vi "o3 Serial Data Recording & DECADEv3.1(serial_sim).vi"() -> ()   [LabVIEW 2014]
uses:
  <vilib>/Platform/TimedLoop/XDataNode/timing_clust.ctl
  <vilib>/Platform/TimedLoop/XDataNode/nitl_modes.ctl
  <vilib>/Platform/TimedLoop/XDataNode/wakeup.ctl
  C:/Program Files (x86)/National Instruments/LabVIEW 2014/examples/Data Communication/Network Streams/Simple Network Streams/support/Network Stream Command.ctl
  <vilib>/Utility/error.llb/whitespace.ctl
  <vilib>/Utility/tcp.llb/UDP Multicast Read-Only Open.vi
  <vilib>/Utility/tcp.llb/UDP Multicast Write-Only Open.vi
  <vilib>/platform/TimedLoop/XDataNode/XDataNode.xnode
  <vilib>/Platform/TimedLoop/XDataNode/XDNodeRunTimeDep.lvlib
  <vilib>/Instr/_visa.llb/VISA Configure Serial Port (Instr).vi
panel:
  out "error out":errorcluster
  out "V6":bool
  in  "Clear Display\nErrors":bool
  out "Data Processing":bool
  out "Serial Visa Error":errorcluster
  out "SEPTIC TCP Error Out":errorcluster
  out "TCP packet\nSend to SEPTIC":bool
  in  "Time Stamp\nOffset":u32=1
  out "UDP_In_Error":errorcluster
  out "UDP_In":string
  out "Data Array":string[](array[string])
  out "UDP packet \nstatus":bool
  out "UDP_Out_Error":errorcluster
  out "FISH TCP Error Out":errorcluster
  out "TCP packet\nSend to FISH":bool
  out "TCP Binary Packet":string
  out "Scan from String Error Counter\nfrom process loop":i32
  out "Read Error Counter\nfrom process loop":i32
  in  "milliseconds to wait":u32=330
  in  "ID":string="±"
  in  "VISA resource name":refnum<visa-resource-name>="ASRL6::INSTR"
  out "Data In Array":string[](array[string])
  out "UDP_ASCII_Out":string
  out "UDP_Pack_num":u32
  in  "Flight Number":string
  in  "aux":string="0"
  in  "inlet_overq_mfm":string="0"
  in  "acs2653pc_hdd":string="0"
  in  "LabviewVIclient vn":string="0"
  in  "LabviewVIserver vn":string="0"
  in  "acs2653pc temp":string="0"
  in  "ue9LJ temp":u16
  in  "PTP Sync":string="0"
  out "Data String":string
  out "Internal packet":string[](array[string])
  out "RAW DATA":string
  in  "stop":bool
  out "Number of Send & Read Error\nfrom Acquire Loop":i32
  out "Command In":string
  # "o3_conc"
  # "Bench_temp"
  # "pressure"
  # "cell_a_nt"
  # "cell_b_int"
  # "flow_a"
  # "flow_b"
  # "lamp_temp"
  # "flags"
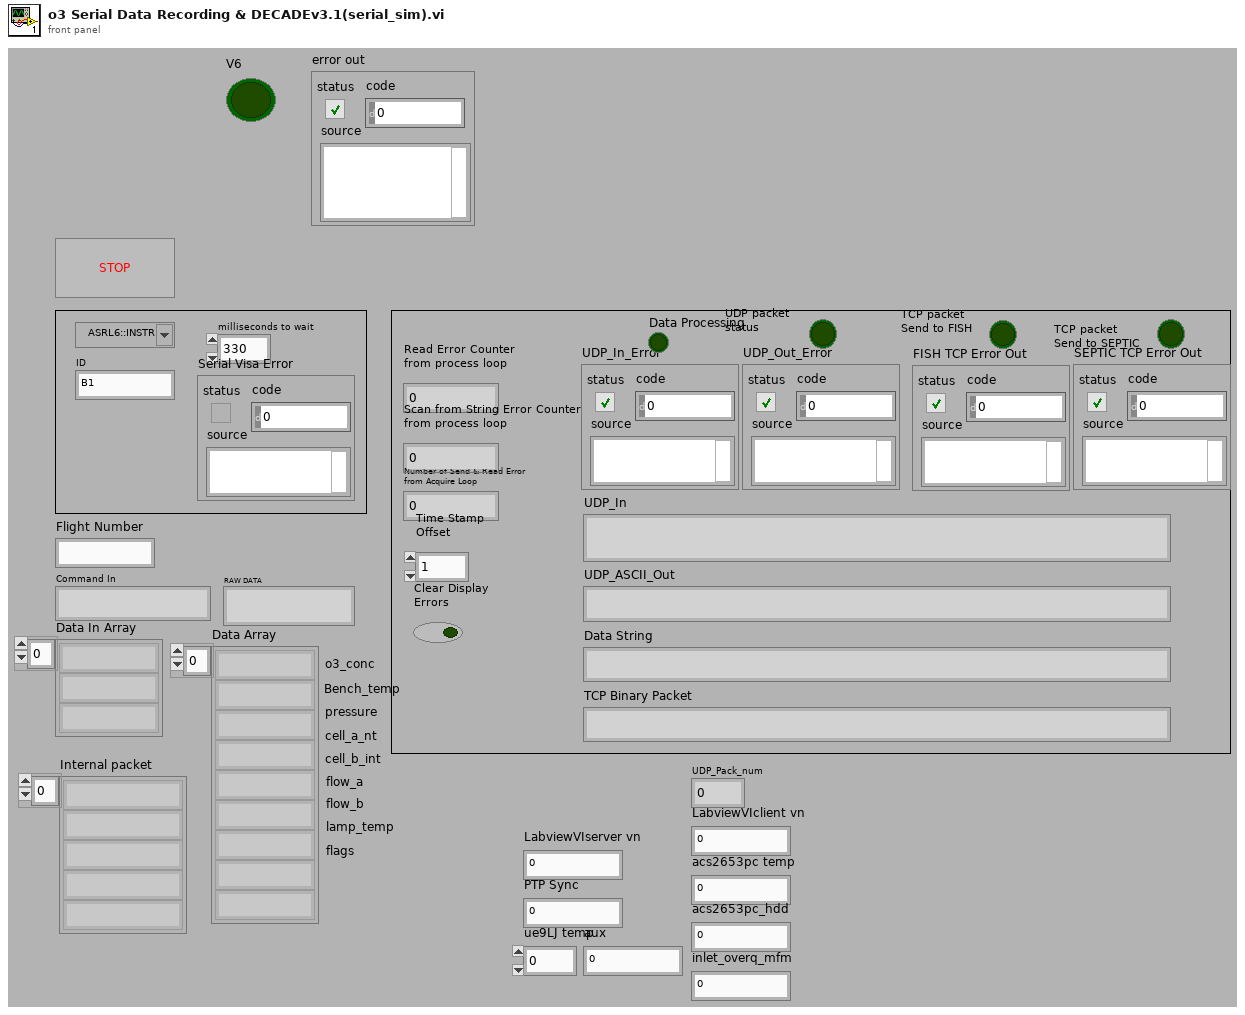
[diagram p1: front panel]
types:
  T1 = typedef "Network Stream Command.ctl" = cluster{"Message":string, "Message Data":variant}
  T2 = typedef "XDNodeRunTimeDep.lvlib/timing_clust.ctl" = cluster{"Expected End [f-1]":u64, "Actual End [f-1]":u64, "Finished Late? [f-1]":bool, "Expected End [i-1]":u64, "Actual End [i-1]":u64, "Finished Late? [i-1]":bool, "Expected Start [i]":u64, "Actual Start [i]":u64, "Expected Start [f]":u64, "Actual Start [f]":u64, "Source Name":string, "Structure Name":string, "Period":i64, "Deadline":i64, "Offset":i64, "Start":i64, "Priority":i32, "Timeout":i32, "Mode":T3, "Wakeup Reason":T4, "Error":errorcluster, "Source Type":string, "Secondary Source Type":string, "Global End Time":u64, "Global Start Time":u64, "Frame Duration":u64, "Iteration Duration":u64, "Assigned CPU":i32, "I/O Scan Engine Mode":u32}
  T3 = typedef "XDNodeRunTimeDep.lvlib/nitl_modes.ctl" = enum32{"No Change", "Process missed periods, maintain original phase", "Discard missed periods, maintain original phase", "Process missed periods, ignore original phase", "Discard missed periods, ignore original phase"}
  T4 = typedef "XDNodeRunTimeDep.lvlib/wakeup.ctl" = enum32{"Normal", "Aborted", "Asynchronous wakeup", "Timing source error", "Timed loop error", "Timeout"}
  T5 = typedef "whitespace.ctl" = u16
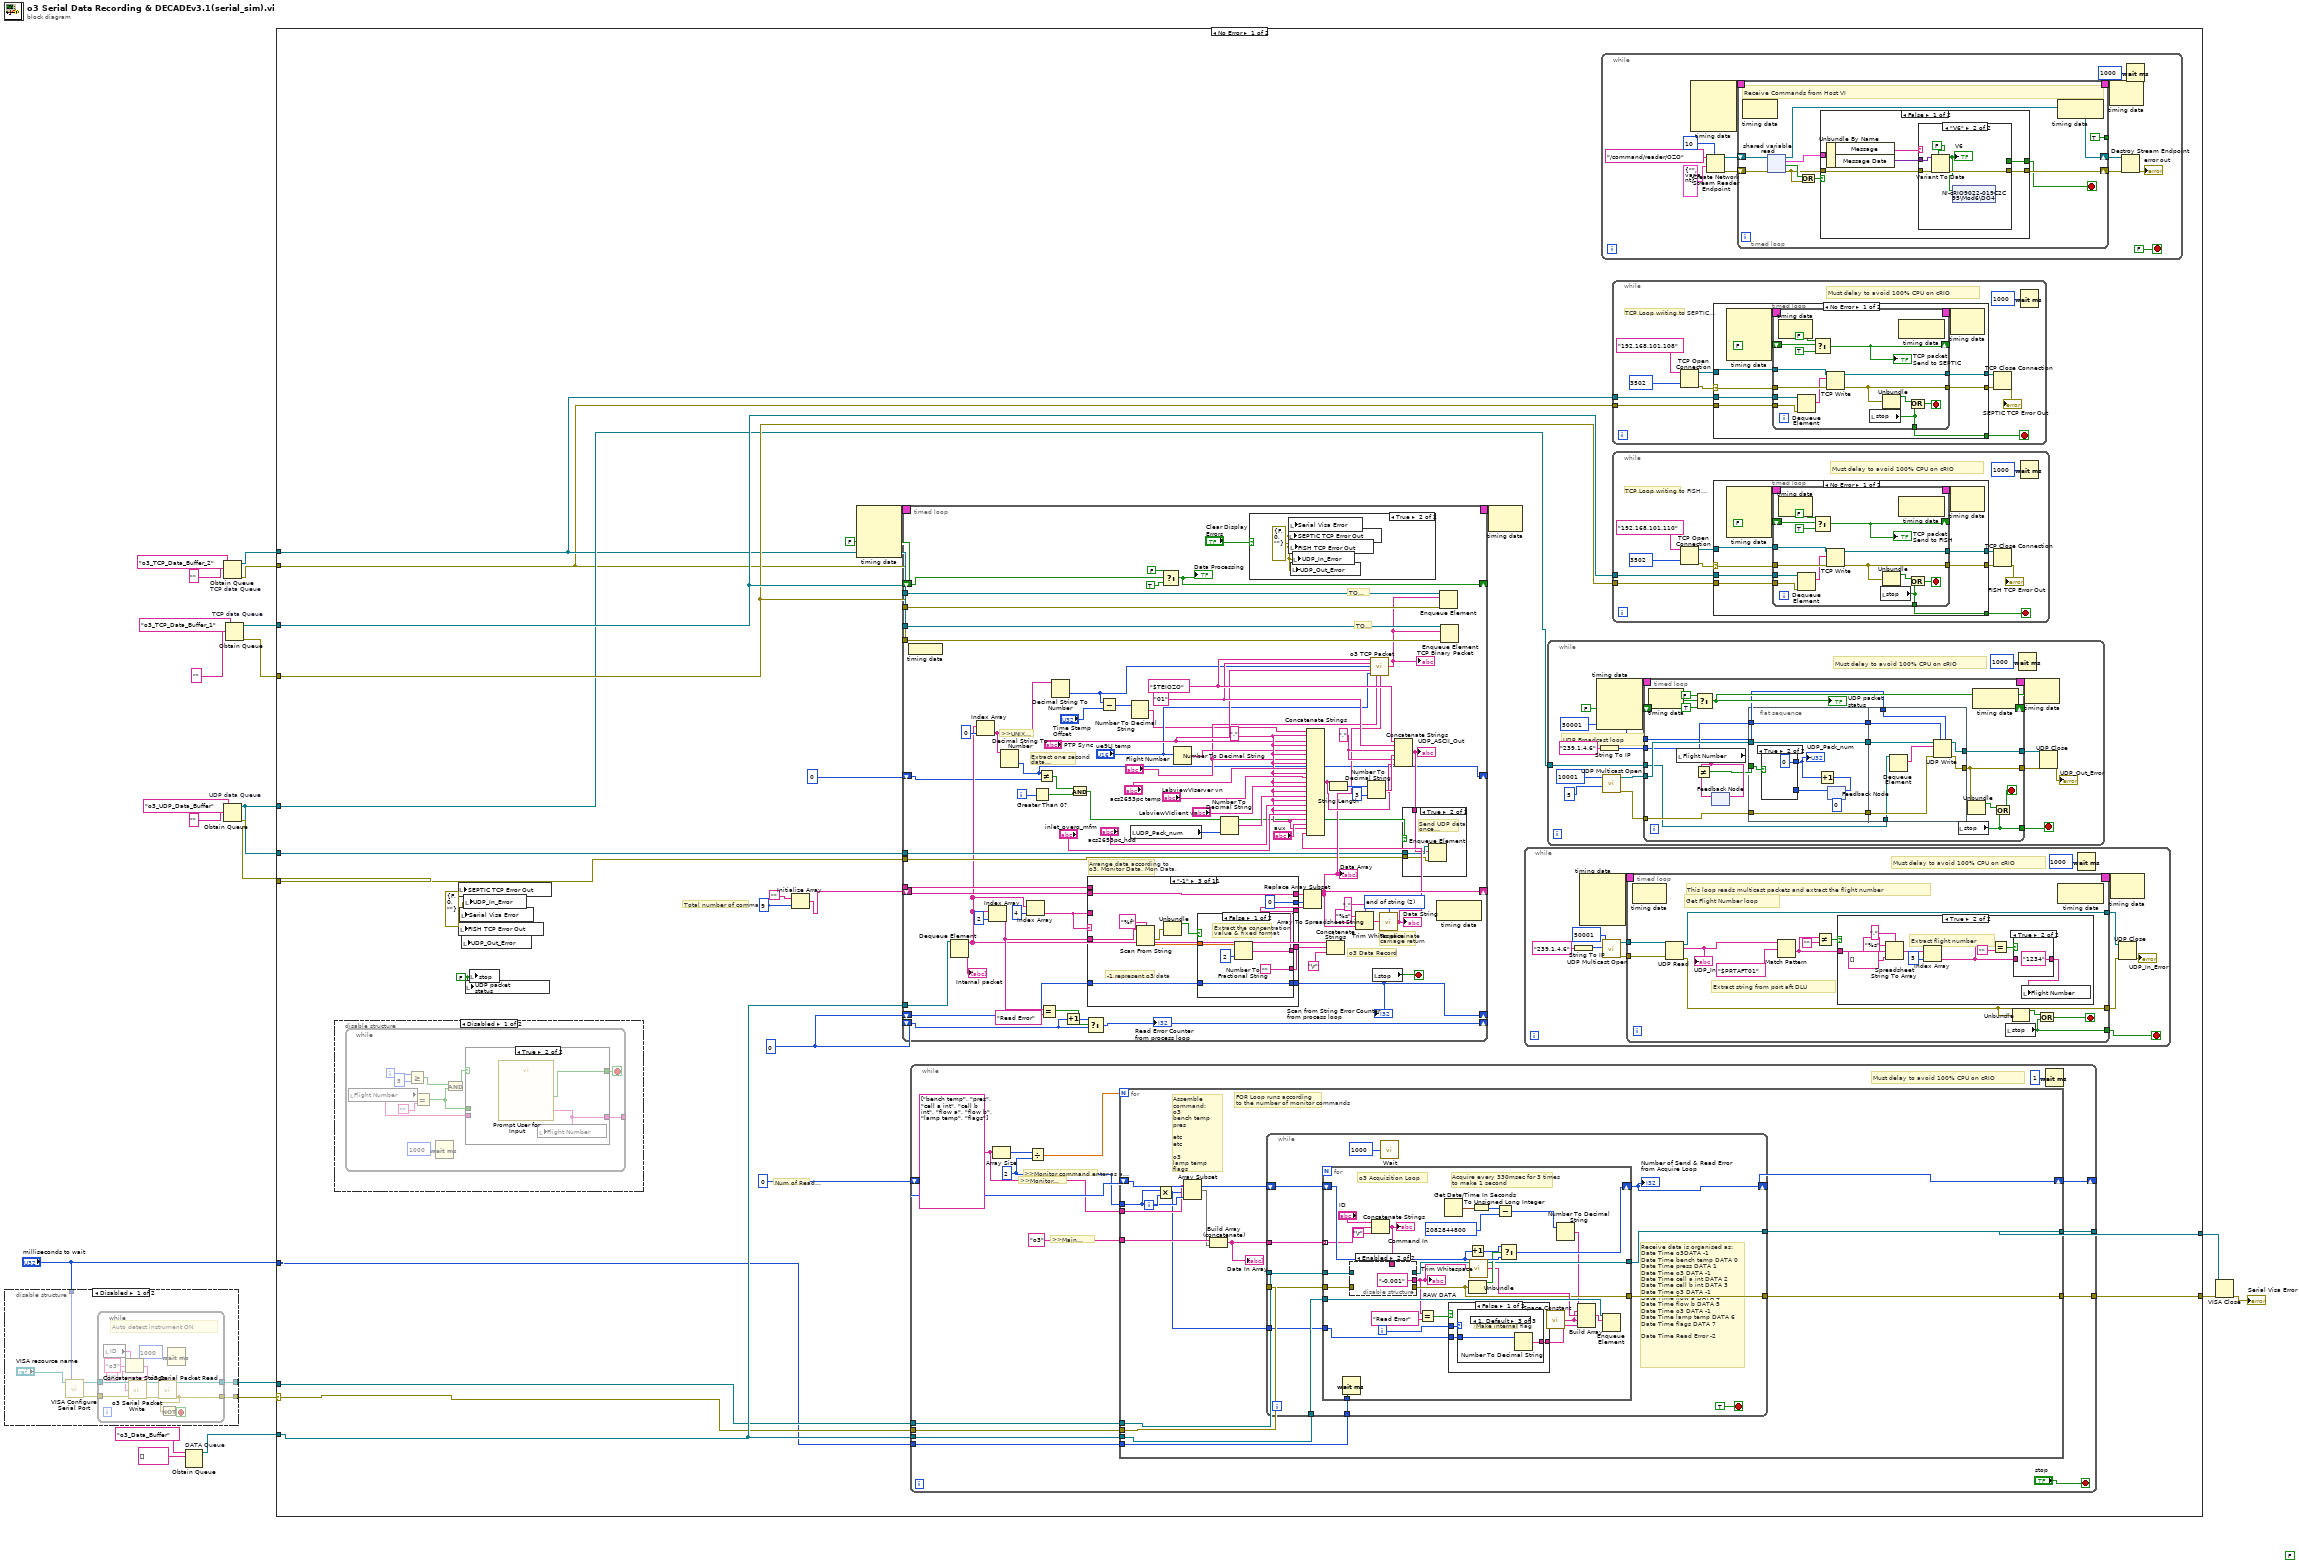
[diagram p0: block diagram]
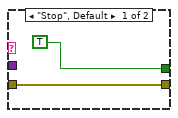
[diagram p3: hidden frame]
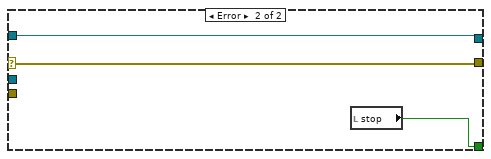
[diagram p7: hidden frame]
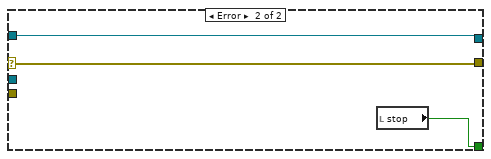
[diagram p8: hidden frame]
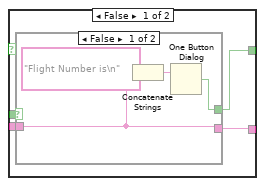
[diagram p9: hidden frame]
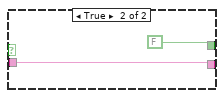
[diagram p10: hidden frame]
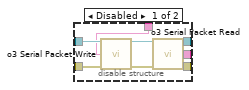
[diagram p13: hidden frame]
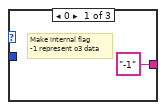
[diagram p14: hidden frame]
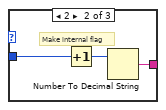
[diagram p15: hidden frame]
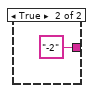
[diagram p16: hidden frame]
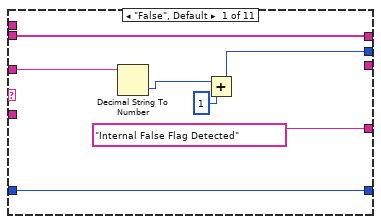
[diagram p19: hidden frame]
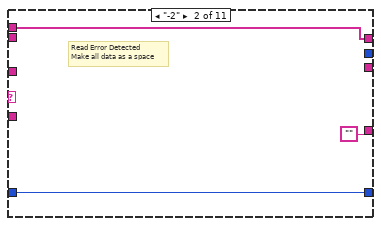
[diagram p20: hidden frame]
diagram:
  (unwired) FALSE
  n1 = disable-structure shown="Disabled" {
    disable-tunnel: "milliseconds to wait" -> [w26 _]
    disable-tunnel: [w25 _] -> w6
    disable-tunnel: [w24 _] -> w5
    frame Disabled {
      n2 = call-poly "VISA Configure Serial Port"("VISA resource name"="VISA resource name", "timeout (10sec)"=w26) -> ("VISA resource name out"=w23:refnum<visa-resource-name>, "error out"=w22:errorcluster)  [unwired: 12 in]
      n3 = while {
        tunnel: [w37] -> w25
        tunnel: [w36] -> w24
        tunnel: w23 -> [w35]
        tunnel: w22 -> [w34]
        stop <- w38 stop-if-true
        # "Auto detect instrument ON"
        n4 = local read "ID"() -> (w32:string)
        n5 = Concatenate Strings(w32, "o3" ("string"), "\r") -> (w29:string)
        n6 = call "o3 Serial Packet Write.vi"("VISA resource name In"=w35, "Data in"=w29, "error in (no error)"=w34) -> ("VISA resource name Out"=w33:refnum<visa-resource-name>, "error out"=w39:errorcluster)  [unwired: 11 in]
        n7 = call "o3 Serial Packet Read.vi"("VISA resource In"=w33, "error in"=w39) -> ("VISA resource Out"=w36:refnum<visa-resource-name>, "error out"=w37:errorcluster)  [unwired: 11 in, 1 out]
        n8 = Not(x=w37) -> (.not. x?=w38:bool)
        n9 = Wait (ms)(milliseconds to wait=u32 1000) -> ()  [unwired: 1 out]
      }
    }
    frame Enabled {
    }
  }
  n10 = Obtain Queue "DATA Queue"(name (unnamed)="o3_Data_Buffer", element data type=string[] []) -> (queue out=w19:refnum<queue>)  [unwired: 3 in, 2 out]
  n11 = Obtain Queue "TCP data Queue"(name (unnamed)="o3_TCP_Data_Buffer_2", element data type="") -> (queue out=w9:refnum<queue>, error out=w8:errorcluster)  [unwired: 3 in, 1 out]
  n12 = Obtain Queue "UDP data Queue"(name (unnamed)="o3_UDP_Data_Buffer", element data type="") -> (queue out=w10:refnum<queue>, error out=w11:errorcluster)  [unwired: 3 in, 1 out]
  n13 = Obtain Queue "TCP data Queue"(name (unnamed)="o3_TCP_Data_Buffer_1", element data type="") -> (queue out=w15:refnum<queue>, error out=w14:errorcluster)  [unwired: 3 in, 1 out]
  n14 = case shown="No Error" w6 {
    selector: w6 -> [w47 w685]
    tunnel: [w63 w685] -> w17
    tunnel: [w62 w684] -> w18
    tunnel: w19 -> [w59 _]
    tunnel: w5 -> [w46 w684]
    tunnel: w15 -> [w52 _]
    tunnel: w14 -> [w51 _]
    tunnel: w10 -> [w50 _]
    tunnel: w11 -> [w49 _]
    tunnel: w10 -> [w48 _]
    tunnel: w9 -> [w44 _]
    tunnel: w8 -> [w43 _]
    tunnel: "milliseconds to wait" -> [w42 _]
    frame No Error {
      w40 = errorcluster {"status"=FALSE, "code"=0, "source"=""} ("UDP Error Out")
      w54 = 0
      w53 = FALSE ("stop")
      # "Num of Read Error"
      # "Total number of commands"
      n15 = disable-structure shown="Disabled" {
        frame Disabled {
          n16 = while {
            tunnel: [w235] -> _
            i -> [w234]
            stop <- w237 stop-if-true
            n17 = local read "Flight Number"() -> (w229:string)
            n18 = Greater Or Equal?(x=w234, y=5) -> (x >= y?=w232:bool)
            n19 = Equal?(x=w229, y="") -> (x = y?=w230:bool)
            n20 = Wait (ms)(milliseconds to wait=u32 1000) -> ()  [unwired: 1 out]
            n21 = And(x=w232, y=w230) -> (x .and. y?=w231:bool)
            n22 = case shown="True" w231 {
              tunnel: [w239 w250] -> w237
              tunnel: [w240 w249] -> w235
              tunnel: w230 -> [w242 _]
              tunnel: w229 -> [w241 _]
              frame False {
                n23 = case shown="False" w242 {
                  tunnel: [w244 w248] -> w240
                  tunnel: w241 -> [w244 w248]
                  tunnel: [w246 FALSE] -> w239
                  frame False {
                    n24 = Concatenate Strings("Flight Number is\n" ("string"), w244) -> (w243:string)
                    n25 = One Button Dialog(message=w243) -> (true=w246:bool)  [unwired: 1 in]
                  }
                  frame True {
                  }
                }
              }
              frame True {
                n26 = call "Prompt User for Input"() -> ("Flight Number BXXX"=w249:string, "OK"=w250:bool)  [unwired: 17 in, 1 out]
                n27 = local write "Flight Number"(w249) -> ()
              }
            }
          }
        }
        frame Enabled {
        }
      }
      n28 = local write "SEPTIC TCP Error Out"(w40) -> ()
      n29 = local write "FISH TCP Error Out"(w40) -> ()
      n30 = local write "Serial Visa Error"(w40) -> ()
      n31 = local write "UDP_Out_Error"(w40) -> ()
      n32 = local write "UDP_In_Error"(w40) -> ()
      n33 = local write "UDP packet \nstatus"(w53) -> ()
      n34 = local write "stop"(w53) -> ()
      n35 = Initialize Array("", 9) -> (w55:string[])
      n36 = node-c288() -> (w61:T2)  [unwired: 4 in]
      n37 = timed-loop {
        timing: w61 -> [_]
        timing-out: [_] -> w60
        tunnel: w59 -> [w469]
        shift-right: [w425] -> _
        shift-left: w55 -> [w450]
        shift-right: [w438] -> _
        shift-left: w54 -> [w435]
        tunnel: w55 -> [w437]
        shift-right: [w433] -> _
        shift-left: w54 -> [w434]
        tunnel: w52 -> [w424]
        tunnel: w51 -> [w423]
        tunnel: w50 -> [w421]
        tunnel: w49 -> [w420]
        shift-right: [w411] -> _
        shift-left: 0 -> [w414]
        tunnel: w44 -> [w409]
        tunnel: w43 -> [w408]
        shift-right: [w399] -> _
        shift-left: FALSE -> [w402]
        i -> [w412]
        stop <- w467 stop-if-true
        w443 = T5 2 items=["both", "start of string", "end of string"] ("location (both)")
        w456 = ","
        w429 = "01"
        w452 = ","
        w430 = "$TEIOZO"
        # "TO SEPTIC"
        # "TO FISH"
        # "Extract one second data\nfor UDP sending"
        # "Arrange data according to\no3, Monitor Data, Mon Data,"
        # "To eliminate\ncarriage return"
        # ">>UNIX TIME>>"
        # "o3 Data Record"
        n38 = node-c288() -> ()  [unwired: 1 in]
        n39 = Dequeue Element(queue=w469) -> (element=w417:string[])  [unwired: 2 in, 3 out]
        "Internal packet" <- w417
        n40 = Index Array(array=w417, index=0) -> (element=w416:string)
        n41 = Index Array(array=w417, index=2) -> (element=w441:string)
        n42 = Decimal String To Number(string=w416) -> (number=w411:i32)  [unwired: 2 in, 1 out]
        n43 = Index Array(array=w417, index=4) -> (element=w449:string)
        n44 = Greater Than 0?(x=w412) -> (x > 0?=w415:bool)
        n45 = Not Equal?(x=w411, y=w414) -> (x != y?=w413:bool)
        n46 = Equal?(x=w441, y="Read Error") -> (x = y?=w439:bool)
        n47 = Decimal String To Number(string=w416) -> (number=w405:i32)  [unwired: 2 in, 1 out]
        n48 = Increment(x=w435) -> (x+1=w436:i32)
        n49 = Compound Arithmetic op=AND(w413, w415) -> (w410:bool)
        n50 = Select(t=w436, s=w439, f=w435) -> (s? t:f=w438:i32)
        "Read Error Counter\nfrom process loop" <- w438
        n51 = case shown="\"-1\"" w449 {
          tunnel: w449 -> [w479 _ _ w515 w537 w559 w581 w603 w625 w647 w669]
          tunnel: w450 -> [w480 _ w494 w516 w538 w560 w582 w604 w626 w648 w670]
          tunnel: w441 -> [_ _ w491 w511 w533 w556 w578 w600 w622 w644 w666]
          tunnel: [w480 w483 w494 w516 w538 w560 w582 w604 w626 w648 w670] -> w448
          tunnel: [w477 _ 0 ("index") w513 w535 w557 w579 w601 w623 w645 w667] -> w447
          tunnel: [_ _ w489 w510 w532 w555 w577 w599 w621 w643 w661] -> w446
          tunnel: w437 -> [_ w483 _ _ _ _ _ _ _ _ _]
          tunnel: w434 -> [w475 w482 w486 w507 w529 w550 w572 w594 w616 w638 w660]
          tunnel: [w475 w482 w485 w506 w528 w549 w571 w593 w615 w637 w659] -> w433
          tunnel: ["Internal False Flag Detected" "" w484 w505 w527 w548 w570 w592 w614 w636 w658] -> w432
          frame "False", Default {
            n52 = Decimal String To Number(string=w479) -> (number=w476:i32)  [unwired: 2 in, 1 out]
            n53 = Add(x=w476, y=1) -> (x+y=w477:i32)
          }
          frame "-2" {
            # "Read Error Detected\nMake all data as a space"
          }
          frame "-1" {
            # "-1 represent o3 data"
            n54 = Scan From String(format string="%f", input string=w491) -> (error out=w488:errorcluster, output 1=w490:dbl)  [unwired: 3 in, 2 out]
            n55 = Unbundle(w488) -> ("status"=w487:bool)  [unwired: 2 out]
            n56 = case shown="False" w487 {
              tunnel: w490 -> [w499 _]
              tunnel: [w498 ""] -> w489
              tunnel: w486 -> [w497 w502]
              tunnel: [w497 w501] -> w485
              tunnel: ["" "Scan from string error"] -> w484
              frame False {
                # "Extract the concentration\nvalue & fixed format"
                n57 = Number To Fractional String(number=w499, precision (6)=i16 2) -> (F-format string=w498:string)  [unwired: 2 in]
              }
              frame True {
                # "If scan from string error,\nreplace data with empty\nstring"
                n58 = Increment(x=w502) -> (x+1=w501:i32)
              }
            }
          }
          frame "0" {
            # "0 represents bench temp data; bench temp 022.6 deg C, actual 022.7"
            n59 = Scan From String(format string="%f ", input string=w511) -> (error out=w509:errorcluster, output 1=w504:dbl)  [unwired: 3 in, 2 out]
            n60 = Decimal String To Number(string=w515) -> (number=w514:i32)  [unwired: 2 in, 1 out]
            n61 = Unbundle(w509) -> ("status"=w508:bool)  [unwired: 2 out]
            n62 = case shown="False" w508 {
              tunnel: w504 -> [w521 _]
              tunnel: [w520 ""] -> w510
              tunnel: w507 -> [w519 w524]
              tunnel: [w519 w523] -> w506
              tunnel: ["" "Scan from string error"] -> w505
              frame False {
                # "Extract the actual value\n& fixed format"
                n63 = Number To Fractional String(number=w521, precision (6)=i16 1) -> (F-format string=w520:string)  [unwired: 2 in]
              }
              frame True {
                # "If scan from string error,\nreplace data with empty\nstring"
                n64 = Increment(x=w524) -> (x+1=w523:i32)
              }
            }
            n65 = Increment(x=w514) -> (x+1=w513:i32)
          }
          frame "1" {
            # "1 represents pres data; pres 725.3 mmHg, actual 725.4"
            n66 = Scan From String(format string="%f ", input string=w533) -> (error out=w531:errorcluster, output 1=w526:dbl)  [unwired: 3 in, 2 out]
            n67 = Decimal String To Number(string=w537) -> (number=w536:i32)  [unwired: 2 in, 1 out]
            n68 = Unbundle(w531) -> ("status"=w530:bool)  [unwired: 2 out]
            n69 = case shown="False" w530 {
              tunnel: w526 -> [w543 _]
              tunnel: [w542 ""] -> w532
              tunnel: w529 -> [w541 w546]
              tunnel: [w541 w545] -> w528
              tunnel: ["" "Scan from string error"] -> w527
              frame False {
                # "Extract the actual value\n& fixed format"
                n70 = Number To Fractional String(number=w543, precision (6)=i16 1) -> (F-format string=w542:string)  [unwired: 2 in]
              }
              frame True {
                # "If scan from string error,\nreplace data with empty\nstring"
                n71 = Increment(x=w546) -> (x+1=w545:i32)
              }
            }
            n72 = Increment(x=w536) -> (x+1=w535:i32)
          }
          frame "2" {
            # "2 represents cell a int data; cell a int 63246 Hz"
            n73 = Scan From String(format string="%f", input string=w556) -> (error out=w552:errorcluster, output 1=w553:dbl)  [unwired: 3 in, 2 out]
            n74 = Decimal String To Number(string=w559) -> (number=w558:i32)  [unwired: 2 in, 1 out]
            n75 = Unbundle(w552) -> ("status"=w551:bool)  [unwired: 2 out]
            n76 = case shown="False" w551 {
              tunnel: [w565 ""] -> w555
              tunnel: w553 -> [w564 _]
              tunnel: w550 -> [w563 w568]
              tunnel: [w563 w567] -> w549
              tunnel: ["" "Scan from string error"] -> w548
              frame False {
                # "Extract the actual value\n& fixed format"
                n77 = Number To Fractional String(number=w564, precision (6)=i16 0) -> (F-format string=w565:string)  [unwired: 2 in]
              }
              frame True {
                # "If scan from string error,\nreplace data with empty\nstring"
                n78 = Increment(x=w568) -> (x+1=w567:i32)
              }
            }
            n79 = Increment(x=w558) -> (x+1=w557:i32)
          }
          frame "3" {
            # "3 represents cell b int data; cell b int 63246 Hz"
            n80 = Scan From String(format string="%f", input string=w578) -> (error out=w574:errorcluster, output 1=w575:dbl)  [unwired: 3 in, 2 out]
            n81 = Decimal String To Number(string=w581) -> (number=w580:i32)  [unwired: 2 in, 1 out]
            n82 = Unbundle(w574) -> ("status"=w573:bool)  [unwired: 2 out]
            n83 = case shown="False" w573 {
              tunnel: [w587 ""] -> w577
              tunnel: w575 -> [w586 _]
              tunnel: w572 -> [w585 w590]
              tunnel: [w585 w589] -> w571
              tunnel: ["" "Scan from string error"] -> w570
              frame False {
                # "Extract the actual value\n& fixed format"
                n84 = Number To Fractional String(number=w586, precision (6)=i16 0) -> (F-format string=w587:string)  [unwired: 2 in]
              }
              frame True {
                # "If scan from string error,\nreplace data with empty\nstring"
                n85 = Increment(x=w590) -> (x+1=w589:i32)
              }
            }
            n86 = Increment(x=w580) -> (x+1=w579:i32)
          }
          frame "4" {
            # "4 represents flow a data; flow a 0.696 l/m"
            n87 = Scan From String(format string="%f", input string=w600) -> (error out=w596:errorcluster, output 1=w597:dbl)  [unwired: 3 in, 2 out]
            n88 = Decimal String To Number(string=w603) -> (number=w602:i32)  [unwired: 2 in, 1 out]
            n89 = Unbundle(w596) -> ("status"=w595:bool)  [unwired: 2 out]
            n90 = case shown="False" w595 {
              tunnel: [w609 ""] -> w599
              tunnel: w597 -> [w608 _]
              tunnel: w594 -> [w607 w612]
              tunnel: [w607 w611] -> w593
              tunnel: ["" "Scan from string error"] -> w592
              frame False {
                # "Extract the actual value\n& fixed format"
                n91 = Number To Fractional String(number=w608, precision (6)=i16 3) -> (F-format string=w609:string)  [unwired: 2 in]
              }
              frame True {
                # "If scan from string error,\nreplace data with empty\nstring"
                n92 = Increment(x=w612) -> (x+1=w611:i32)
              }
            }
            n93 = Increment(x=w602) -> (x+1=w601:i32)
          }
          frame "5" {
            # "5 represents flow b data; flow b 0.696 l/m"
            n94 = Scan From String(format string="%f", input string=w622) -> (error out=w618:errorcluster, output 1=w619:dbl)  [unwired: 3 in, 2 out]
            n95 = Decimal String To Number(string=w625) -> (number=w624:i32)  [unwired: 2 in, 1 out]
            n96 = Unbundle(w618) -> ("status"=w617:bool)  [unwired: 2 out]
            n97 = case shown="False" w617 {
              tunnel: [w631 ""] -> w621
              tunnel: w619 -> [w630 _]
              tunnel: w616 -> [w629 w634]
              tunnel: [w629 w633] -> w615
              tunnel: ["" "Scan from string error"] -> w614
              frame False {
                # "Extract the actual value\n& fixed format"
                n98 = Number To Fractional String(number=w630, precision (6)=i16 3) -> (F-format string=w631:string)  [unwired: 2 in]
              }
              frame True {
                # "If scan from string error,\nreplace data with empty\nstring"
                n99 = Increment(x=w634) -> (x+1=w633:i32)
              }
            }
            n100 = Increment(x=w624) -> (x+1=w623:i32)
          }
          frame "6" {
            # "6 represents lamp temp data; lamp temp 056.1 deg C"
            n101 = Scan From String(format string="%f", input string=w644) -> (error out=w640:errorcluster, output 1=w641:dbl)  [unwired: 3 in, 2 out]
            n102 = Decimal String To Number(string=w647) -> (number=w646:i32)  [unwired: 2 in, 1 out]
            n103 = Unbundle(w640) -> ("status"=w639:bool)  [unwired: 2 out]
            n104 = case shown="False" w639 {
              tunnel: [w653 ""] -> w643
              tunnel: w641 -> [w652 _]
              tunnel: w638 -> [w651 w656]
              tunnel: [w651 w655] -> w637
              tunnel: ["" "Scan from string error"] -> w636
              frame False {
                # "Extract the actual value\n& fixed format"
                n105 = Number To Fractional String(number=w652, precision (6)=i16 1) -> (F-format string=w653:string)  [unwired: 2 in]
              }
              frame True {
                # "If scan from string error,\nreplace data with empty\nstring"
                n106 = Increment(x=w656) -> (x+1=w655:i32)
              }
            }
            n107 = Increment(x=w646) -> (x+1=w645:i32)
          }
          frame "7" {
            # "7 represents flags data; flags 1c100000"
            n108 = Scan From String(format string="%f", input string=w666) -> (error out=w664:errorcluster, output 1=w662:dbl)  [unwired: 3 in, 2 out]
            n109 = Decimal String To Number(string=w669) -> (number=w668:i32)  [unwired: 2 in, 1 out]
            n110 = Unbundle(w664) -> ("status"=w663:bool)  [unwired: 2 out]
            n111 = case shown="False" w663 {
              tunnel: w662 -> [w672 _]
              tunnel: [w671 ""] -> w661
              tunnel: w660 -> [w675 w678]
              tunnel: [w675 w677] -> w659
              tunnel: ["" "Scan from string error"] -> w658
              frame False {
                # "Extract the actual value\n& fixed format"
                n112 = Number To Fractional String(number=w672, precision (6)=i16 1) -> (F-format string=w671:string)  [unwired: 2 in]
              }
              frame True {
                # "If scan from string error,\nreplace data with empty\nstring"
                n113 = Increment(x=w678) -> (x+1=w677:i32)
              }
            }
            n114 = Increment(x=w668) -> (x+1=w667:i32)
          }
        }
        "Scan from String Error Counter\nfrom process loop" <- w433
        n115 = Subtract(x=w405, y="Time Stamp\nOffset") -> (x-y=w406:u32)
        n116 = local read "UDP_Pack_num"() -> (w461:u32)
        n117 = Number To Decimal String(number=w406) -> (decimal integer string=w403:string)  [unwired: 1 in]
        n118 = Select(t=FALSE, s=w402, f=TRUE) -> (s? t:f=w399:bool)
        "Data Processing" <- w399
        n119 = Number To Decimal String(number="ue9LJ temp") -> (decimal integer string=w431:string)  [unwired: 1 in]
        n120 = Number To Decimal String(number=w461) -> (decimal integer string=w460:string)  [unwired: 1 in]
        n121 = case shown="True" "Clear Display\nErrors" {
          frame False {
          }
          frame True {
            w470 = errorcluster {"status"=FALSE, "code"=0, "source"=""} ("UDP Error Out")
            n122 = local write "SEPTIC TCP Error Out"(w470) -> ()
            n123 = local write "Serial Visa Error"(w470) -> ()
            n124 = local write "FISH TCP Error Out"(w470) -> ()
            n125 = local write "UDP_Out_Error"(w470) -> ()
            n126 = local write "UDP_In_Error"(w470) -> ()
          }
        }
        n127 = Replace Array Subset(array=w448, new element=w446, index=w447) -> (w425:string[])
        "Data Array" <- w425
        n128 = Concatenate Strings(w417, w432, "\r") -> ()  [unwired: 1 out]
        n129 = Array To Spreadsheet String(delimiter (Tab)=",", array=w425, 3:"%s" ("format string")) -> (spreadsheet string=w442:string)
        n130 = call "o3 TCP Packet.vi"("ID"=w430, "Version"=w429, "utc_time"=w405, "PTP Sync"="PTP Sync", "ue9LJ temp"="ue9LJ temp", "Flight Number"="Flight Number", "Data Array"=w425) -> ("TCP Binary Packet"=w407:string)  [unwired: 8 in]
        "TCP Binary Packet" <- w407
        n131 = local read "stop"() -> (w467:bool)
        n132 = call <vilib>:"Trim Whitespace.vi"("string"=w442, "location (both)"=w443) -> ("trimmed string"=w422:string)
        "Data String" <- w422
        n133 = Concatenate Strings(w403, w456, "PTP Sync", w456, w431, w456, "Flight Number", w456, "acs2653pc temp", w456, "LabviewVIserver vn", w456, "LabviewVIclient vn", w456, w460, w456, "acs2653pc_hdd", w456, "inlet_overq_mfm", w456, "aux", w456, w422) -> (w451:string)
        n134 = String Length(string=w451) -> (length=w455:i32)
        n135 = Number To Decimal String(number=w455, width (-)=i16 3) -> (decimal integer string=w453:string)
        n136 = Concatenate Strings(w430, w429, w452, w453, w452, w451) -> (w419:string)
        "UDP_ASCII_Out" <- w419
        n137 = case shown="True" w410 {
          tunnel: w421 -> [_ w473]
          tunnel: w420 -> [_ w472]
          tunnel: w419 -> [_ w471]
          frame False {
          }
          frame True {
            # "Send UDP data once\na second"
            n138 = Enqueue Element(queue=w473, element=w471, error in (no error)=w472) -> ()  [unwired: 1 in, 3 out]
          }
        }
        n139 = node-c288() -> ()  [unwired: 1 in, 1 out]
        n140 = Enqueue Element(queue=w409, element=w407, error in (no error)=w408) -> ()  [unwired: 1 in, 3 out]
        n141 = Enqueue Element(queue=w424, element=w407, error in (no error)=w423) -> ()  [unwired: 1 in, 3 out]
      }
      n142 = while {
        tunnel: [w312] -> w63
        tunnel: w46 -> [w323]
        tunnel: w47 -> [w322]
        tunnel: [w321] -> w62
        tunnel: w59 -> [w320]
        shift-right: [w318] -> _
        shift-left: 0 -> [w319]
        tunnel: w42 -> [w310]
        stop <- "stop" stop-if-true
        w313 = 2
        w315 = string[] ["bench temp", "pres", "cell a int", "cell b int", "flow a", "flow b", "lamp temp", "flags"]
        # "Must delay to avoid 100% CPU on cRIO"
        # ">>Monitor command enter as a pair>>"
        # ">>Main commands>>"
        # ">>Monitor Command>>"
        n143 = Array Size(array=w315) -> (size(s)=w316:i32)
        n144 = Divide(x=w316, y=w313) -> (x/y=w314:dbl)
        n145 = for {
          N: w314 -> [_]
          tunnel: w323 -> [w331]
          tunnel: w322 -> [w330]
          tunnel: [w338] -> w312
          shift-right: [w336] -> w318
          shift-left: w319 -> [w337]
          tunnel: [w335] -> w321
          tunnel: w320 -> [w334]
          tunnel: w315 -> [w327]
          tunnel: "o3" -> [w332]
          tunnel: w313 -> [w328]
          tunnel: w310 -> [w324]
          i -> [w329]
          # "FOR Loop runs according\nto the number of monitor commands"
          # "Assemble command:\no3\nbench temp\npres\n\netc\netc\n\no3\nlamp temp\nflags"
          n146 = Multiply(x=w328, y=w329) -> (x*y=w325:i32)
          n147 = Array Subset(array=w327, index=w325, length=w328) -> (w326:string[])
          n148 = Build Array (concatenate)(w332, w326) -> (w333:string[])
          "Data In Array" <- w333
          n149 = while {
            tunnel: [w350] -> w338
            tunnel: w333 -> [w348]
            tunnel: [w346] -> w335
            tunnel: w334 -> [w345]
            tunnel: w330 -> [w344]
            tunnel: w331 -> [w343]
            tunnel: w325 -> [w342]
            shift-right: [w347] -> w336
            shift-left: w337 -> [w349]
            tunnel: w324 -> [w339]
            stop <- TRUE stop-if-true
            # "Receive data is organised as:\nDate Time o3DATA -1\nDate Time bench temp DATA 0\nDate Time press DATA 1\nDate Time o3 DATA -1\nDate Time cell a int DATA 2\nDate Time cell b int DATA 3\nDate Time o3 DATA -1\nDate Time flow a DATA 4\nDate Time flow b DATA 5\nDate Time o3 DATA -1\nDate Time lamp temp DATA 6\nDate Time flags DATA 7\n\nDate Time Read Error -2"
            n150 = for {
              tunnel: w344 -> [w367]
              tunnel: [w368] -> w350
              tunnel: w348 -> [w365] mode=indexing
              tunnel: [w369] -> w346
              tunnel: w345 -> [w373]
              tunnel: w343 -> [w370]
              tunnel: w342 -> [w364]
              shift-right: [w377] -> w347
              shift-left: w349 -> [w378]
              tunnel: w339 -> [w353]
              i -> [w357]
              # "Acquire every 330msec for 3 times\nto make 1 second"
              # "o3 Acquisition Loop"
              n151 = Wait (ms)(milliseconds to wait=w353) -> ()  [unwired: 1 out]
              n152 = Concatenate Strings("ID", w365, "\r") -> (w363:string)
              "Command In" <- w363
              n153 = disable-structure shown="Enabled" {
                disable-tunnel: w370 -> [w384 _]
                disable-tunnel: [w383 _] -> w369
                disable-tunnel: [w382 _] -> w368
                disable-tunnel: w367 -> [w381 _]
                disable-tunnel: w363 -> [w380 _]
                disable-tunnel: [w379 "-0.001" ("RAW DATA")] -> w360
                frame Disabled {
                  n154 = call "o3 Serial Packet Write.vi"("VISA resource name In"=w384, "Data in"=w380, "error in (no error)"=w381) -> ("VISA resource name Out"=w386:refnum<visa-resource-name>, "error out"=w385:errorcluster)  [unwired: 11 in]
                  n155 = call "o3 Serial Packet Read.vi"("VISA resource In"=w386, "error in"=w385) -> ("VISA resource Out"=w383:refnum<visa-resource-name>, "Data Out"=w379:string, "error out"=w382:errorcluster)  [unwired: 11 in]
                }
                frame Enabled {
                }
              }
              "RAW DATA" <- w360
              n156 = Equal?(x=w360, y="Read Error") -> (x = y?=w358:bool)
              n157 = Get Date/Time In Seconds() -> (seconds since 1Jan1904=w352:timestamp)
              n158 = case shown="False" w358 {
                tunnel: [w390 "-2"] -> w371
                tunnel: w357 -> [w389 _]
                tunnel: w364 -> [w388 _]
                frame False {
                  n159 = case shown="1, Default" w389 {
                    tunnel: ["-1" w394 w396] -> w390
                    tunnel: w388 -> [_ w392 w395]
                    frame 0 {
                      # "Make internal flag\n-1 represent o3 data"
                    }
                    frame 2 {
                      # "Make internal flag"
                      n160 = Increment(x=w392) -> (x+1=w393:i32)
                      n161 = Number To Decimal String(number=w393) -> (decimal integer string=w394:string)  [unwired: 1 in]
                    }
                    frame 1, Default {
                      # "Make internal flag"
                      n162 = Number To Decimal String(number=w395) -> (decimal integer string=w396:string)  [unwired: 1 in]
                    }
                  }
                }
                frame True {
                }
              }
              n163 = Increment(x=w378) -> (x+1=w374:i32)
              n164 = Unbundle(w368) -> ("status"=w375:bool)  [unwired: 2 out]
              n165 = call <vilib>:"Trim Whitespace.vi"("string"=w360) -> ("trimmed string"=w372:string)  [unwired: 1 in]
              n166 = To Unsigned Long Integer(number=w352) -> (unsigned 32bit integer=w356:u32)
              n167 = Subtract(x=w356, y=u32 2082844800) -> (x-y=w351:u32)
              n168 = Select(t=w374, s=w375, f=w378) -> (s? t:f=w377:i32)
              n169 = call <vilib>:"Space Constant.vi"() -> ("String"=w361:string)
              n170 = Number To Decimal String(number=w351) -> (decimal integer string=w354:string)  [unwired: 1 in]
              n171 = Build Array(w354, w361, w372, w361, w371) -> (w362:string[])
              n172 = Enqueue Element(queue=w373, element=w362) -> ()  [unwired: 2 in, 3 out]
            }
            "Number of Send & Read Error\nfrom Acquire Loop" <- w347
            n173 = call "Wait"("Count(mSec)"=u32 1000) -> ()  [unwired: 1 out]
          }
        }
        n174 = Wait (ms)(milliseconds to wait=u32 1) -> ()  [unwired: 1 out]
      }
      n175 = node-c288(w60) -> ()  [unwired: 1 out]
      n176 = while {
        stop <- w109 stop-if-true
        # "Must delay to avoid 100% CPU on cRIO"
        n177 = String To IP(1:"239.1.4.6" ("name")) -> (0:w116:u32)
        n178 = node-c288() -> (w107:T2)  [unwired: 4 in]
        n179 = call-poly <vilib>:"UDP Multicast Open.vi"("multicast addr"=w116, "port"=u16 50001) -> ("error out"=w112:errorcluster, "connection ID"=w113:refnum<k16>)  [unwired: 7 in, 1 out]
        n180 = timed-loop {
          tunnel: w113 -> [w128]
          tunnel: w112 -> [w127]
          tunnel: [w122] -> w111
          tunnel: [w120] -> w110
          tunnel: [w118] -> w109
          timing: w107 -> [_]
          timing-out: [_] -> w106
          stop <- w119 stop-if-true
          # "Extract string from port aft DLU"
          # "Get Flight Number loop"
          # "This loop reads multicast packets and extract the flight number"
          n181 = node-c288() -> ()  [unwired: 1 in, 1 out]
          n182 = UDP Read(connection ID=w128, 8:w127) -> (data out=w123:string, error out=w120:errorcluster, 3:w122:refnum<k16>)  [unwired: 2 in, 2 out]
          "UDP_In" <- w123
          n183 = Match Pattern(string=w123, regular expression="$PRTAFT01") -> (after substring=w124:string)  [unwired: 1 in, 3 out]
          n184 = Not Equal?(x=w124, y="") -> (x != y?=w125:bool)
          n185 = case shown="True" w125 {
            tunnel: w124 -> [_ w135]
            frame False {
            }
            frame True {
              # "Extract flight number"
              n186 = Spreadsheet String To Array(delimiter (Tab)=",", format string="%s", spreadsheet string=w135, array type (2D Dbl)=string[] []) -> (array=w137:string[])
              n187 = Index Array(array=w137, index=5) -> (element=w132:string)
              n188 = Equal?(x=w132, y="") -> (x = y?=w134:bool)
              n189 = case shown="True" w134 {
                tunnel: [w141 "1234"] -> w131
                tunnel: w132 -> [w141 _]
                frame False {
                }
                frame True {
                }
              }
              n190 = local write "Flight Number"(w131) -> ()
            }
          }
          n191 = local read "stop"() -> (w118:bool)
          n192 = Unbundle(w120) -> ("status"=w121:bool)  [unwired: 2 out]
          n193 = Compound Arithmetic op=OR(w121, w118) -> (w119:bool)
          n194 = node-c288() -> ()  [unwired: 1 in, 1 out]
        }
        n195 = Wait (ms)(milliseconds to wait=u32 1000) -> ()  [unwired: 1 out]
        n196 = node-c288(w106) -> ()  [unwired: 1 out]
        n197 = UDP Close(connection ID=w111, 8:w110) -> (error out=→"UDP_In_Error":errorcluster)  [unwired: 1 out]
      }
      n198 = while {
        tunnel: w48 -> [w252]
        stop <- w253 stop-if-true
        # "Must delay to avoid 100% CPU on cRIO"
        # "UDP Broadcast loop"
        n199 = node-c288() -> (w255:T2)  [unwired: 4 in]
        n200 = String To IP(1:"239.1.4.6" ("name")) -> (0:w257:u32)
        n201 = call-poly <vilib>:"UDP Multicast Open.vi"("time-to-live (1)"=u16 5, "port"=u16 10001) -> ("error out"=w265:errorcluster, "connection ID"=w266:refnum<k16>)  [unwired: 8 in]
        n202 = timed-loop {
          tunnel: w266 -> [w286]
          tunnel: w265 -> [w285]
          tunnel: [w272] -> w261
          shift-right: [w275] -> _
          shift-left: FALSE -> [w278]
          tunnel: [w270] -> w259
          tunnel: w257 -> [w274]
          tunnel: u16 50001 ("port or service name") -> [w273]
          timing: w255 -> [_]
          timing-out: [_] -> w254
          tunnel: [w268] -> w253
          tunnel: w252 -> [w267]
          stop <- w269 stop-if-true
          n203 = node-c288() -> ()  [unwired: 1 in, 1 out]
          n204 = local read "Flight Number"() -> (w281:string)
          n205 = Select(t=FALSE, s=w278, f=TRUE) -> (s? t:f=w275:bool)
          "UDP packet \nstatus" <- w275
          n206 = feedback-in #1(w281) -> ()
          n207 = feedback #1() -> (w280:string)  [unwired: 1 in]
          n208 = Not Equal?(x=w281, y=w280) -> (x != y?=w279:bool)
          n209 = flat-sequence {
            tunnel: w274 -> [w294]
            tunnel: w285 -> [w295]
            tunnel: w286 -> [w296]
            tunnel: [w296] -> w284
            tunnel: [w295] -> w283
            tunnel: [w294] -> w282
            tunnel: w279 -> [w293]
            tunnel: w273 -> [w306]
            tunnel: w284 -> [w305]
            tunnel: w283 -> [w304]
            tunnel: w282 -> [w303]
            tunnel: [w302] -> w272
            tunnel: [w301] -> w270
            tunnel: w267 -> [w300]
            frame #0 {
              n210 = feedback #2(u32 0) -> (w290:u32)
              n211 = case shown="True" w293 {
                tunnel: w290 -> [w297 _]
                tunnel: [w297 u32 0] -> w289
                frame False {
                }
                frame True {
                }
              }
              "UDP_Pack_num" <- w289
              n212 = Increment(x=w289) -> (x+1=w291:u32)
              n213 = feedback-in #2(w291) -> ()
            }
            frame #1 {
              n214 = Dequeue Element(queue=w300) -> (element=w299:string)  [unwired: 2 in, 3 out]
              n215 = UDP Write(address=w303, port or service name=w306, connection ID=w305, data in=w299, 8:w304) -> (error out=w301:errorcluster, 3:w302:refnum<k16>)  [unwired: 1 in]
            }
          }
          n216 = local read "stop"() -> (w268:bool)
          n217 = Unbundle(w270) -> ("status"=w271:bool)  [unwired: 2 out]
          n218 = node-c288() -> ()  [unwired: 1 in, 1 out]
          n219 = Compound Arithmetic op=OR(w271, w268) -> (w269:bool)
        }
        n220 = Wait (ms)(milliseconds to wait=u32 1000) -> ()  [unwired: 1 out]
        n221 = node-c288(w254) -> ()  [unwired: 1 out]
        n222 = UDP Close(connection ID=w261, 8:w259) -> (error out=→"UDP_Out_Error":errorcluster)  [unwired: 1 out]
      }
      n223 = while {
        stop <- FALSE stop-if-true
        n224 = node-c288() -> (w65:T2)  [unwired: 4 in]
        n225 = Create Network Stream Reader Endpoint(7:10 ("reader buffer size"), 9:T1 {"Message"="", "Message Data"=variant} ("Message Cluster"), 11:"/command/reader/OZO" ("reader url")) -> (0:w71:errorcluster, 3:w72:refnum<k21>)  [unwired: 4 in]
        n226 = timed-loop "Host->Target Command Reader" {
          shift-right: [w82] -> w69
          shift-left: w71 -> [w85]
          shift-right: [w83] -> w68
          shift-left: w72 -> [w84]
          tunnel: [TRUE] -> _
          timing: w65 -> [_]
          timing-out: [_] -> w64
          stop <- w76 stop-if-true
          # "Receive Commands from Host VI"
          n227 = node-c288() -> ()  [unwired: 1 in, 1 out]
          n228 = shared-variable-read(w84, w85) -> (w83:refnum<k21>, w78:errorcluster, w80:bool, w81:T1)  [unwired: 1 in]
          n229 = Or(x=w80, y=w78) -> (x .or. y?=w79:bool)
          n230 = case shown="False" w79 {
            selector: w79 -> [_ w101]
            tunnel: w78 -> [w93 w102]
            tunnel: [w92 w102] -> w82
            tunnel: w81 -> [w90 _]
            tunnel: [w91 w101] -> w76
            frame False {
              n231 = Unbundle By Name(w90) -> ("Message"=w89:string, "Message Data"=w88:variant)
              n232 = case shown="\"V6\"" w89 {
                tunnel: w93 -> [w95 w100]
                tunnel: [w95 w99] -> w92
                tunnel: w88 -> [_ w98]
                tunnel: [TRUE _] -> w91
                frame "Stop", Default {
                }
                frame "V6" {
                  n233 = Variant To Data(error in=w100, type=FALSE, Variant=w98) -> (data=w96:bool, error out=w99:errorcluster)
                  "V6" <- w96
                  n234 = shared-variable "NI-cRIO9022-019C2C95\\Mod6\\DO4"(w96) -> ()  [unwired: 1 in, 1 out]
                }
              }
            }
            frame True {
            }
          }
          n235 = node-c288() -> ()  [unwired: 1 in, 1 out]
        }
        n236 = node-c288(w64) -> ()  [unwired: 1 out]
        n237 = Destroy Stream Endpoint(8:w69, 11:w68) -> (0:→"error out":errorcluster)
        n238 = Wait (ms)(milliseconds to wait=u32 1000) -> ()  [unwired: 1 out]
      }
      n239 = while {
        tunnel: w43 -> [w147]
        tunnel: w44 -> [w146]
        stop <- w150 stop-if-true
        # "Must delay to avoid 100% CPU on cRIO"
        # "TCP Loop writing to SEPTIC Tank"
        n240 = TCP Open Connection(address="192.168.101.108", remote port or service name=u16 3502) -> (connection ID=w153:refnum<k5>, error out=w148:errorcluster)  [unwired: 3 in]
        n241 = case shown="No Error" w148 {
          selector: w148 -> [w158 w185]
          tunnel: w153 -> [w163 w186]
          tunnel: [w162 w186] -> w152
          tunnel: [w161 w185] -> w151
          tunnel: [w160 w184] -> w150
          tunnel: w146 -> [w157 _]
          tunnel: w147 -> [w156 _]
          frame No Error {
            n242 = node-c288() -> (w165:T2)  [unwired: 4 in]
            n243 = timed-loop {
              tunnel: w163 -> [w179]
              tunnel: w158 -> [w178]
              tunnel: [w177] -> w162
              tunnel: [w176] -> w161
              tunnel: [w166] -> w160
              shift-right: [w170] -> _
              shift-left: FALSE -> [w173]
              timing: w165 -> [_]
              timing-out: [_] -> w164
              tunnel: w157 -> [w169]
              tunnel: w156 -> [w168]
              stop <- w174 stop-if-true
              n244 = node-c288() -> ()  [unwired: 1 in, 1 out]
              n245 = Dequeue Element(queue=w169, error in (no error)=w168) -> (element=w167:string)  [unwired: 1 in, 3 out]
              n246 = Select(t=FALSE, s=w173, f=TRUE) -> (s? t:f=w170:bool)
              "TCP packet\nSend to SEPTIC" <- w170
              n247 = TCP Write(connection ID=w179, data in=w167, error in (no error)=w178) -> (connection ID out=w177:refnum<k5>, error out=w176:errorcluster)  [unwired: 1 in, 1 out]
              n248 = local read "stop"() -> (w166:bool)
              n249 = Unbundle(w176) -> ("status"=w175:bool)  [unwired: 2 out]
              n250 = node-c288() -> ()  [unwired: 1 in, 1 out]
              n251 = Compound Arithmetic op=OR(w175, w166) -> (w174:bool)
            }
            n252 = node-c288(w164) -> ()  [unwired: 1 out]
          }
          frame Error {
            n253 = local read "stop"() -> (w184:bool)
          }
        }
        n254 = TCP Close Connection(connection ID=w152, error in (no error)=w151) -> (error out=→"SEPTIC TCP Error Out":errorcluster)  [unwired: 1 in, 1 out]
        n255 = Wait (ms)(milliseconds to wait=u32 1000) -> ()  [unwired: 1 out]
      }
      n256 = while {
        tunnel: w52 -> [w189]
        tunnel: w51 -> [w188]
        stop <- w192 stop-if-true
        # "Must delay to avoid 100% CPU on cRIO"
        # "TCP Loop writing to FISH Tank"
        n257 = TCP Open Connection(address="192.168.101.110", remote port or service name=u16 3502) -> (connection ID=w195:refnum<k5>, error out=w190:errorcluster)  [unwired: 3 in]
        n258 = case shown="No Error" w190 {
          selector: w190 -> [w200 w227]
          tunnel: w195 -> [w205 w228]
          tunnel: [w204 w228] -> w194
          tunnel: [w203 w227] -> w193
          tunnel: [w202 w226] -> w192
          tunnel: w189 -> [w199 _]
          tunnel: w188 -> [w198 _]
          frame No Error {
            n259 = node-c288() -> (w207:T2)  [unwired: 4 in]
            n260 = timed-loop {
              tunnel: w205 -> [w221]
              tunnel: w200 -> [w220]
              tunnel: [w219] -> w204
              tunnel: [w218] -> w203
              tunnel: [w215] -> w202
              shift-right: [w211] -> _
              shift-left: FALSE -> [w214]
              timing: w207 -> [_]
              timing-out: [_] -> w206
              tunnel: w199 -> [w210]
              tunnel: w198 -> [w209]
              stop <- w216 stop-if-true
              n261 = node-c288() -> ()  [unwired: 1 in, 1 out]
              n262 = Dequeue Element(queue=w210, error in (no error)=w209) -> (element=w208:string)  [unwired: 1 in, 3 out]
              n263 = Select(t=FALSE, s=w214, f=TRUE) -> (s? t:f=w211:bool)
              "TCP packet\nSend to FISH" <- w211
              n264 = TCP Write(connection ID=w221, data in=w208, error in (no error)=w220) -> (connection ID out=w219:refnum<k5>, error out=w218:errorcluster)  [unwired: 1 in, 1 out]
              n265 = local read "stop"() -> (w215:bool)
              n266 = Unbundle(w218) -> ("status"=w217:bool)  [unwired: 2 out]
              n267 = node-c288() -> ()  [unwired: 1 in, 1 out]
              n268 = Compound Arithmetic op=OR(w217, w215) -> (w216:bool)
            }
            n269 = node-c288(w206) -> ()  [unwired: 1 out]
          }
          frame Error {
            n270 = local read "stop"() -> (w226:bool)
          }
        }
        n271 = TCP Close Connection(connection ID=w194, error in (no error)=w193) -> (error out=→"FISH TCP Error Out":errorcluster)  [unwired: 1 in, 1 out]
        n272 = Wait (ms)(milliseconds to wait=u32 1000) -> ()  [unwired: 1 out]
      }
    }
    frame Error {
    }
  }
  n273 = VISA Close(VISA resource name=w18, error in (no error)=w17) -> (error out=→"Serial Visa Error":errorcluster)
